vi "LoadUnflattenClassData.vi"(8 "error in":errorcluster, 10 "Class Data File Path":path, 11 "VeriStandTestCase in":refnum<class "VeriStandTestCase.lvclass">) -> (0 "error out":errorcluster, 3 "VeriStandTestCase out":refnum<class "VeriStandTestCase.lvclass">)   [LabVIEW 2027, in "VeriStandTestCase.lvclass"]
uses:
  VeriStandTestCase.lvclass
  VeriStandTestUtilities/VeriStandTestUtilities.lvlib
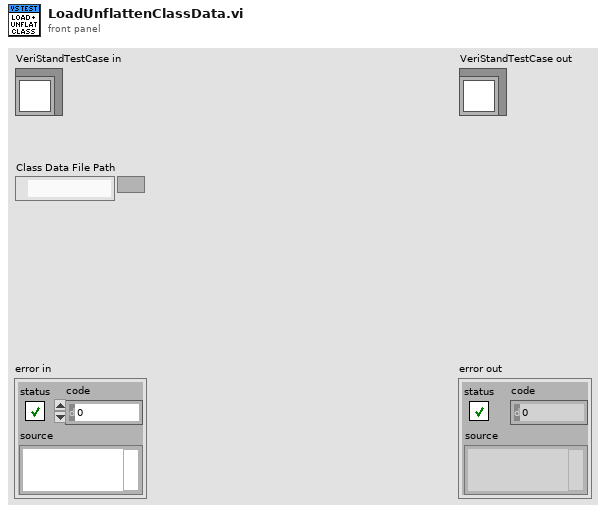
[diagram p1: front panel]
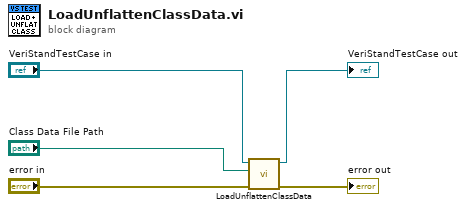
[diagram p0: block diagram]
diagram:
  n1 = call "LoadUnflattenClassData.vi"("error in"="error in", "Class Data File Path"="Class Data File Path", "TestCase in"="VeriStandTestCase in") -> ("error out"=→"error out":errorcluster, "TestCase out"=→"VeriStandTestCase out":refnum<class "VeriStandTestCase.lvclass">)  [unwired: 7 in]
